vi "Write Time Stamp - Time Stamp.vi"(8 "error in (no error)":errorcluster, 10 "time stamp":timestamp, 11 "NT Base in":refnum<class "NT Base.lvclass">) -> (0 "error out":errorcluster, 3 "NT Base out":refnum<class "NT Base.lvclass">)   [LabVIEW 2020, in "PV Access.lvlib" / "PV Data.lvlib" / "NT Base.lvclass"]
uses:
  NT Base.lvclass
  NT Base.lvclass/NT Base.ctl
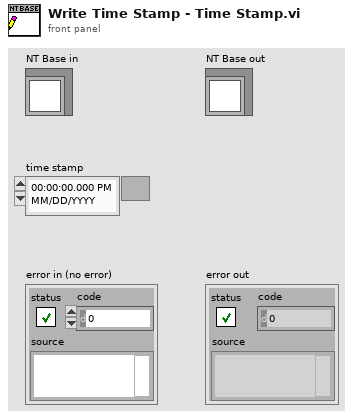
[diagram p1: front panel]
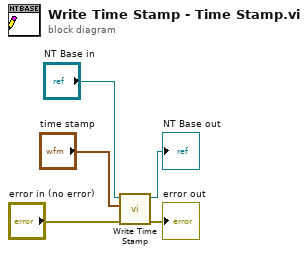
[diagram p0: block diagram]
diagram:
  n1 = call-dynamic "Write Time Stamp.vi"("error in"="error in (no error)", "time stamp"="time stamp", "Has Timestamp in"="NT Base in") -> ("error out"=→"error out":errorcluster, "Has Timestamp out"=→"NT Base out":refnum<class "NT Base.lvclass">)  [unwired: 7 in]
